vi "SetRAMValveState.vi"(7 "Timeout (ms)":u32=2000, 8 "Error In":errorcluster, 10 "Valve State":T1, 11 "Sierra M100 In":refnum<visa-resource-name>) -> (0 "Error Out":errorcluster, 2 "Set?":bool, 3 "Sierra M100 Out":refnum<visa-resource-name>)   [LabVIEW 2012, in "Sierra-M100.lvlib"]
doc: "This VI sets the valve state in random access memory (RAM). RAM is volatile and the valve state will NOT be retained during power cycling. Use \"Set Flash Valve State\" VI instead."
uses:
  Sierra-M100.lvlib
  Controls/ValveState.ctl
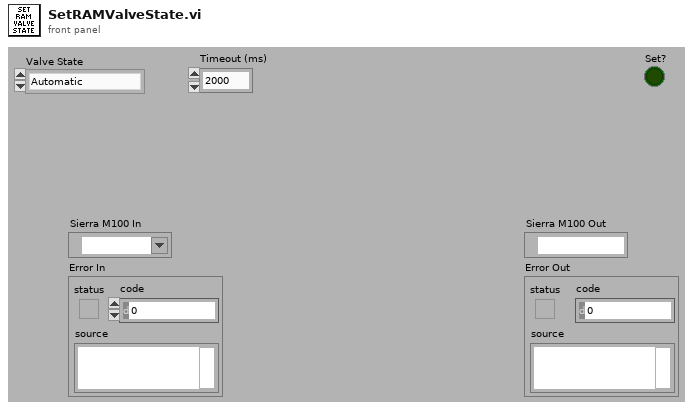
[diagram p1: front panel]
types:
  T1 = typedef "Sierra-M100.lvlib/ValveState.ctl" = enum16{"Automatic", "Closed", "Purge"}
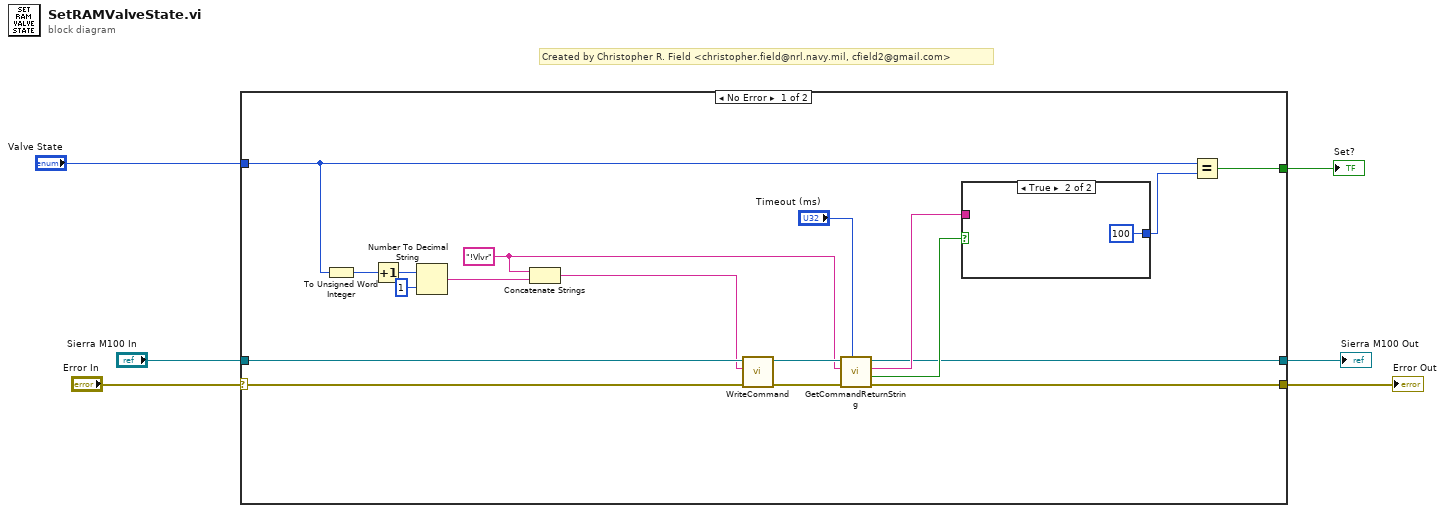
[diagram p0: block diagram]
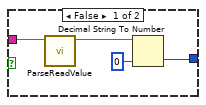
[diagram p2: hidden frame]
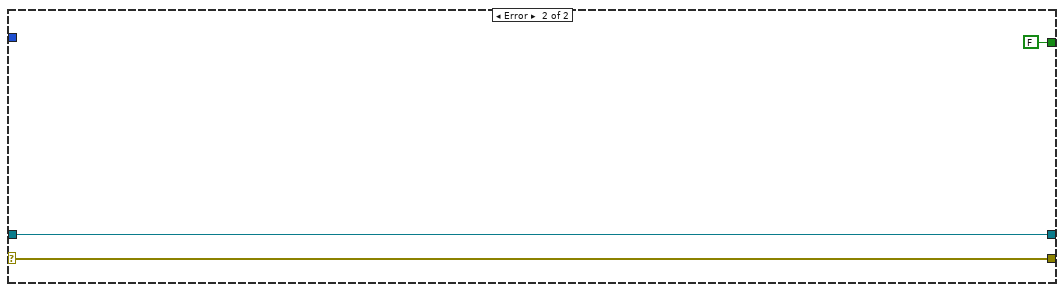
[diagram p3: hidden frame]
diagram:
  # "Created by Christopher R. Field <christopher.field@nrl.navy.mil, cfield2@gmail.com>"
  n1 = case shown="No Error" "Error In" {
    selector: "Error In" -> [w7 w31]
    tunnel: [w16 FALSE] -> w6
    tunnel: "Sierra M100 In" -> [w15 w32]
    tunnel: [w11 w32] -> w4
    tunnel: [w10 w31] -> w3
    tunnel: "Valve State" -> [w9 _]
    frame No Error {
      w14 = "!Vlvr"
      n2 = To Unsigned Word Integer(number=w9) -> (unsigned 16bit integer=w22:u16)
      n3 = Increment(x=w22) -> (x+1=w21:u16)
      n4 = Number To Decimal String(number=w21, width (-)=i16 1) -> (decimal integer string=w24:string)
      n5 = Concatenate Strings(w14, w24) -> (w8:string)
      n6 = call "WriteCommand.vi"("Error In"=w7, "Command"=w8, "Sierra M100 In"=w15) -> ("Error Out"=w19:errorcluster, "Sierra M100 Out"=w20:refnum<visa-resource-name>)  [unwired: 5 in, 2 out]
      n7 = call "GetCommandReturnString.vi"("Timeout (ms)"="Timeout (ms)", "Error In"=w19, "Command"=w14, "Sierra M100 In"=w20) -> ("Error Out"=w10:errorcluster, "Timeout?"=w13:bool, "Return String"=w12:string, "Sierra M100 Out"=w11:refnum<visa-resource-name>)  [unwired: 4 in]
      n8 = case shown="True" w13 {
        tunnel: [w25 u16 100] -> w17
        tunnel: w12 -> [w28 _]
        frame False {
          n9 = call "ParseReadValue.vi"("Read Buffer"=w28) -> ("Value"=w27:string)  [unwired: 10 in]
          n10 = Decimal String To Number(string=w27, default (0L)=u16 0 ("default (0 I32)")) -> (number=w25:u16)  [unwired: 1 in, 1 out]
        }
        frame True {
        }
      }
      n11 = Equal?(x=w9, y=w17) -> (x = y?=w16:bool)
    }
    frame Error {
    }
  }
  "Sierra M100 Out" <- w4
  "Error Out" <- w3
  "Set?" <- w6
